vi "_TEST_ObjCacher2.vi"() -> ()   [LabVIEW 2017]
panel:
  in  "String":string[](array[string])=["", "abc"]
  in  "loop":i32=1000
  out "ms":u32[](array[numeric])
  # "比较效率"
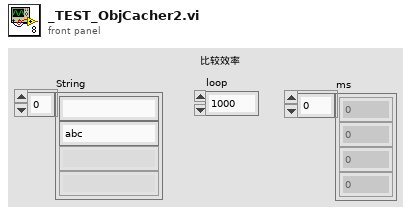
[diagram p1: front panel]
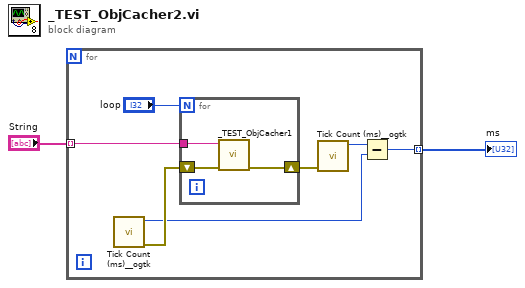
[diagram p0: block diagram]
diagram:
  n1 = for {
    tunnel: [w4] -> w2 mode=indexing
    tunnel: "String" -> [w3] mode=indexing
    n2 = call <userlib>:"Tick Count (ms)__ogtk.vi"() -> ("error out"=w8:errorcluster, "millisecond timer value"=w5:u32)  [unwired: 10 in]
    n3 = for {
      N: "loop" -> [_]
      shift-right: [w11] -> w7
      shift-left: w8 -> [w12]
      tunnel: w3 -> [w10]
      n4 = call "_TEST_ObjCacher1.vi"("error in (no error)"=w12, "String"=w10) -> ("error out"=w11:errorcluster)  [unwired: 9 in]
    }
    n5 = call <userlib>:"Tick Count (ms)__ogtk.vi"("error in (no error)"=w7) -> ("millisecond timer value"=w6:u32)  [unwired: 9 in, 1 out]
    n6 = Subtract(x=w6, y=w5) -> (x-y=w4:u32)
  }
  "ms" <- w2
